vi "analyseMatlab.vi"(8 "error in (no error)":errorcluster, 10 "Array":T1(array[cluster]), 11 "FluorescenceAnalyser in":refnum<class "FluorescenceAnalyser.lvclass">) -> (0 "error out":errorcluster, 3 "FluorescenceAnalyser out":refnum<class "FluorescenceAnalyser.lvclass">)   [LabVIEW 2011, in "Tools.lvlib" / "Imaging.lvlib" / "FluorescenceAnalyser.lvclass"]
uses:
  FluorescenceAnalyser.lvclass
  Filing/FileNeologist/FileNeologist.lvclass
  ImageAnalyser.lvclass
  Filing/FileSystem/FileSystem.lvclass
  Imaging.lvlib
panel:
  out "laserMinMax":dbl[](array[numeric])
  out "atomMinMax":dbl[](array[numeric])
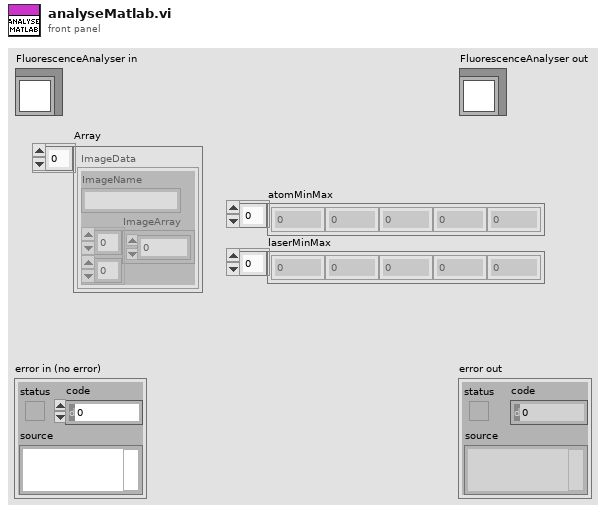
[diagram p1: front panel]
types:
  T1 = cluster{"ImageName":string, "ImageArray":dbl[][]}[]
  T2 = cluster{"Name":string, "Results":dbl[], "AnalysisType":string}
  T3 = cluster{"Left":i32, "Top":i32, "Right":i32, "Bottom":i32}
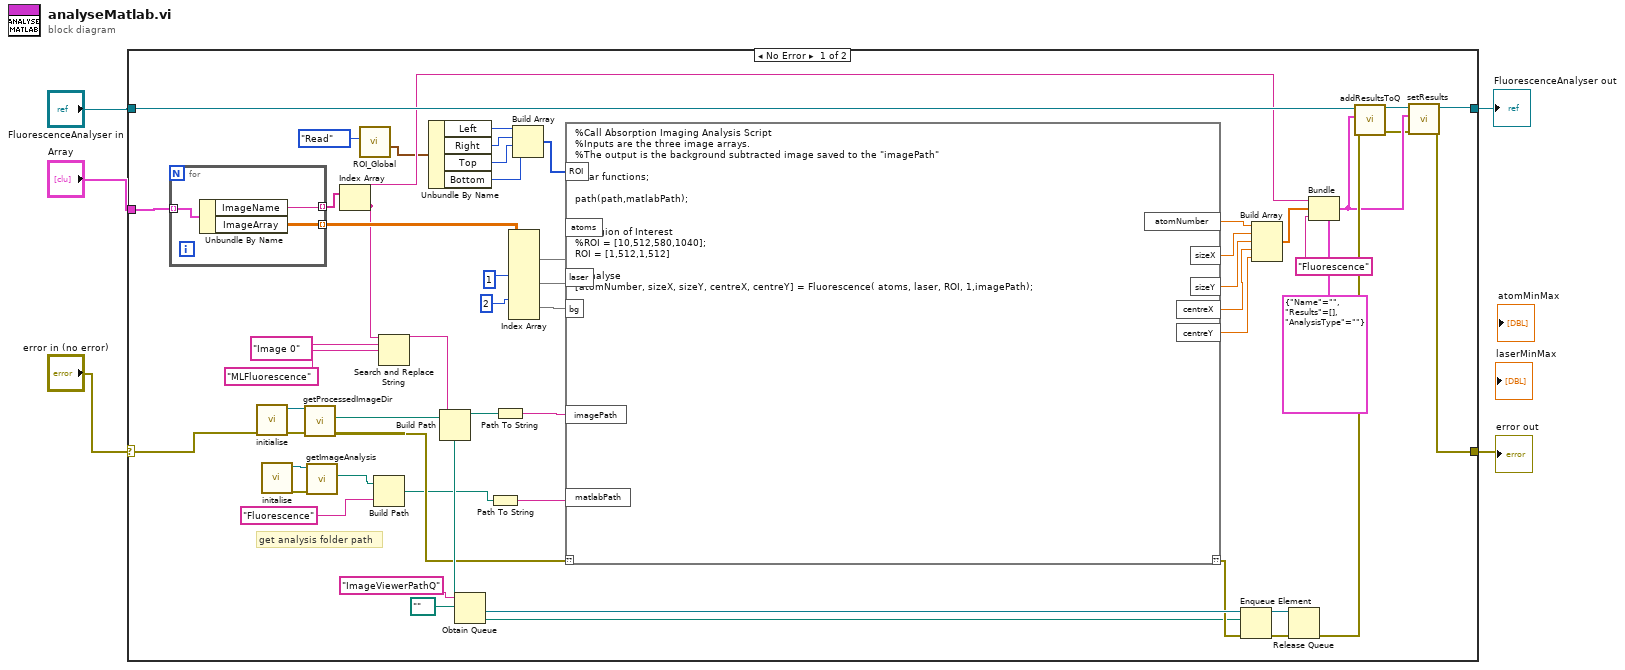
[diagram p0: block diagram]
diagram:
  n1 = case shown="No Error" "error in (no error)" {
    selector: "error in (no error)" -> [w31 w63]
    tunnel: [w19 w63] -> w2
    tunnel: [w22 w62] -> w1
    tunnel: "FluorescenceAnalyser in" -> [w57 w62]
    tunnel: "Array" -> [w56 _]
    frame No Error {
      # "get analysis folder path"
      n2 = for {
        tunnel: w56 -> [w61] mode=indexing
        tunnel: [w60] -> w55 mode=indexing
        tunnel: [w59] -> w51 mode=indexing
        n3 = Unbundle By Name(w61) -> ("ImageName"=w59:string, "ImageArray"=w60:dbl[][])
      }
      n4 = call "initialise.vi"("error in (no error)"=w31) -> ("error out"=w47:errorcluster, "FileNeologist out"=w48:refnum<class "FileNeologist.lvclass">)  [unwired: 9 in]
      n5 = call "initalise.vi"() -> ("error out"=w27:errorcluster, "FileSystem out"=w28:refnum<class "FileSystem.lvclass">)  [unwired: 10 in]
      n6 = call-dynamic "getProcessedImageDir.vi"("error in (no error)"=w47, "FileNeologist in"=w48) -> ("error out"=w30:errorcluster, "Path"=w46:path)  [unwired: 7 in, 1 out]
      n7 = call "getImageAnalysis.vi"("error in (no error)"=w27, "FileSystem in"=w28) -> ("ImageAnalysis"=w26:path)  [unwired: 7 in, 2 out]
      n8 = Index Array(array=w51) -> (element=w34:string)  [unwired: 1 in]
      n9 = call "ROI_Global.vi"("Action"=enum16{"Write", "Read"}."Read") -> ("ROI"=w14:T3)  [unwired: 10 in]
      n10 = Build Path(base path=w26, name or relative path="Fluorescence") -> (appended path=w24:path)
      n11 = Search and Replace String(input string=w34, search string="Image 0", replace string="MLFluorescence") -> (result string=w45:string)  [unwired: 5 in, 3 out]
      n12 = Unbundle By Name(w14) -> ("Left"=w12:i32, "Right"=w11:i32, "Top"=w10:i32, "Bottom"=w9:i32)
      n13 = Build Path(base path=w46, name or relative path=w45) -> (appended path=w37:path)
      n14 = Obtain Queue(name (unnamed)="ImageViewerPathQ", element data type=path "") -> (queue out=w42:refnum<queue>)  [unwired: 3 in, 2 out]
      n15 = Path To String(path=w24) -> (string=w29:string)
      n16 = Path To String(path=w37) -> (string=w39:string)
      n17 = Index Array(array=w55, index (dim 0) #2=1, index (dim 0) #3=2) -> (element #1=w15:dbl[][], element #2=w53:dbl[][], element #3=w52:dbl[][])  [unwired: 7 in]
      n18 = Build Array(w12, w11, w10, w9) -> (w8:i32[])
      n19 = script code="%Call Absorption Imaging Analysis Script \n%Inputs are the three image arrays.\n%The output is the background subtracted image saved to the \"imagePath\"\n\nclear functions;\n\npath(path,matlabPath);\n\n\n% Region of Interest\n%ROI = [10,512,580,1040];\nROI = [1,512,1,512]\n\n%Analyse\n[atomNumber, sizeX, sizeY, centreX, centreY] = Fluorescence( atoms, laser, ROI, 1,imagePath);"("??"=w30, "bg"=w52, "laser"=w53, "atoms"=w15, "imagePath"=w39, "matlabPath"=w29, "ROI"=w8) -> ("??"=w38:errorcluster, "atomNumber"=w18:dbl, "sizeX"=w17:dbl, "sizeY"=w16:dbl, "centreX"=w7:dbl, "centreY"=w6:dbl)
      n20 = Enqueue Element(queue=w42, element=w37, error in (no error)=w38) -> (queue out=w41:refnum<queue>, error out=w40:errorcluster)  [unwired: 1 in, 1 out]
      n21 = Build Array(w18, w17, w16, w7, w6) -> (w35:dbl[])
      n22 = Release Queue(queue=w41, error in (no error)=w40) -> (error out=w36:errorcluster)  [unwired: 1 in, 2 out]
      n23 = Bundle(cluster=T2 {"Name"="", "Results"=[], "AnalysisType"=""} ("output cluster"), "Name"=w34, "Results"=w35, "AnalysisType"="Fluorescence") -> (w21:T2)
      n24 = call "addResultsToQ.vi"("error in (no error)"=w36, "Results"=w21, "ImageAnalyser in"=w57) -> ("error out"=w20:errorcluster, "ImageAnalyser out"=w23:refnum<class "FluorescenceAnalyser.lvclass">)  [unwired: 7 in]
      n25 = call "setResults.vi"("error in (no error)"=w20, "results"=w21, "ImageAnalyser in"=w23) -> ("error out"=w19:errorcluster, "ImageAnalyser out"=w22:refnum<class "FluorescenceAnalyser.lvclass">)  [unwired: 7 in]
    }
    frame Error {
    }
  }
  "error out" <- w2
  "FluorescenceAnalyser out" <- w1
